vi "Set Items (Label).vi"(6 "Items":refnum<class "IObject.lvclass">[](array[class]), 8 "error in (no error)":errorcluster, 10 "Label":string, 11 "MMI Scaling in":refnum<class "IContainer.lvclass">) -> (0 "error out":errorcluster, 2 "Match?":bool, 3 "MMI Scaling out":refnum<class "IContainer.lvclass">, 5 "Old items":refnum<class "IObject.lvclass">[](array[class]))   [LabVIEW 2013, in "IContainer.lvclass"]
doc: "Copyright 2018, Wiebe Walstra, wiebe@carya.nl."
uses:
  IContainer.lvclass
  IObject.lvclass
  IContainer.lvclass/IContainer.ctl
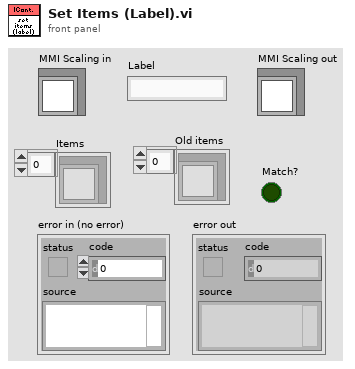
[diagram p1: front panel]
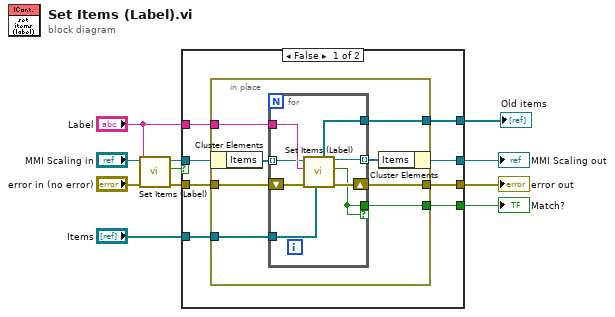
[diagram p0: block diagram]
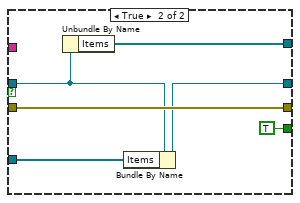
[diagram p2: hidden frame]
diagram:
  n1 = call-parent "Set Items (Label).vi"("error in (no error)"="error in (no error)", "Label"="Label", "MMI Scaling in"="MMI Scaling in") -> ("error out"=w5:errorcluster, "Match?"=w3:bool, "MMI Scaling out"=w8:refnum<class "IContainer.lvclass">)  [unwired: 5 in, 1 out]
  n2 = case shown="False" w3 {
    tunnel: [w19 w41] -> w11
    tunnel: [w18 w39] -> w10
    tunnel: w8 -> [w17 w38]
    tunnel: "Label" -> [w16 _]
    tunnel: w5 -> [w15 w41]
    tunnel: [w14 TRUE ("Match?")] -> w4
    tunnel: "Items" -> [w12 w37]
    tunnel: [w13 w36] -> w1
    frame False {
      n3 = in-place {
        in-place-border: [w27] -> w19
        in-place-border: w15 -> [w26]
        in-place-border: w16 -> [w25]
        in-place-border: [w22] -> w14
        in-place-border: [w21] -> w13
        in-place-border: w12 -> [w20]
        n4 = in-place-cluster #1(w17) -> ("Items"=w24:refnum<class "IObject.lvclass">[])
        n5 = for {
          tunnel: [w34] -> w23 mode=indexing
          tunnel: w24 -> [w31] mode=indexing
          shift-right: [w35] -> w27
          shift-left: w26 -> [w32]
          tunnel: w25 -> [w33]
          tunnel: [w30] -> w22 if=w30
          tunnel: [w29] -> w21
          tunnel: w20 -> [w28]
          n6 = call-dynamic "Set Items (Label).vi"("Items"=w28, "error in (no error)"=w32, "Label"=w33, "MMI Scaling in"=w31) -> ("error out"=w35:errorcluster, "Match?"=w30:bool, "MMI Scaling out"=w34:refnum<class "IObject.lvclass">, "Old items"=w29:refnum<class "IObject.lvclass">[])  [unwired: 4 in]
        }
        n7 = in-place-cluster #1("Items"=w23) -> (w18:refnum<class "IContainer.lvclass">)
      }
    }
    frame True {
      n8 = Unbundle By Name(w38) -> ("Items"=w36:refnum<class "IObject.lvclass">[])
      n9 = Bundle By Name(cluster=w38, "Items"=w37) -> (w39:refnum<class "IContainer.lvclass">)
    }
  }
  "error out" <- w11
  "MMI Scaling out" <- w10
  "Match?" <- w4
  "Old items" <- w1
